vi "FPGA_Write.vi"(5 "Value":u32 format="%x", 7 "Offset":u32, 8 "Error_In":errorcluster, 11 "VISA_Rsrc_In":refnum<visa-resource-name>) -> (0 "Error_Out":errorcluster, 3 "VISA_Rsrc_Out":refnum<visa-resource-name>)   [LabVIEW 2018]
uses:
  <vilib>/Instr/_visa.llb/VISA Register Access Address Space.ctl
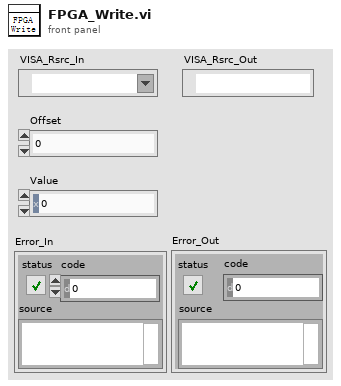
[diagram p1: front panel]
types:
  T1 = typedef "VISA Register Access Address Space.ctl" = u16
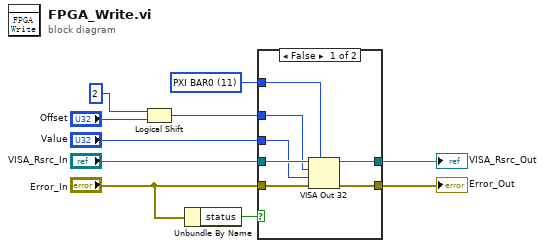
[diagram p0: block diagram]
diagram:
  w1 = T1 11 items=["VXI/VME A16"=1, "VXI/VME A24"=2, "VXI/VME A32"=3, "VXI/VME A64"=4, "PXI Memory Allocations"=9, "PXI Configuration"=10, "PXI BAR0"=11, "PXI BAR1"=12, "PXI BAR2"=13, "PXI BAR3"=14, "PXI BAR4"=15, "PXI BAR5"=16] ("Address Space")
  n1 = Logical Shift(y=i16 2, x="Offset") -> (x << y=w4:u32)
  n2 = Unbundle By Name("Error_In") -> ("status"=w3:bool)
  n3 = case shown="False" w3 {
    tunnel: "Error_In" -> [w17 w18]
    tunnel: "VISA_Rsrc_In" -> [w16 w19]
    tunnel: "Value" -> [w15 _]
    tunnel: [w14 w19] -> w7
    tunnel: [w13 w18] -> w2
    tunnel: w4 -> [w12 _]
    tunnel: w1 -> [w11 _]
    frame False {
      n4 = VISA Out 32(7:w11, 8:w17, 9:w15, 10:w12, 11:w16) -> (0:w13:errorcluster, 3:w14:refnum<visa-resource-name>)
    }
    frame True {
    }
  }
  "VISA_Rsrc_Out" <- w7
  "Error_Out" <- w2
